vi "Controller Test Bench (11).vi"() -> ()   [LabVIEW 2022 SP3]
uses:
  WhiteNoise.ctl
  <vilib>/sound2/lvsound2.llb/Sound Data Format.ctl
  <vilib>/Utility/error.llb/DialogType.ctl
  <vilib>/sound2/lvsound2.llb/Sampling Mode.ctl
  <vilib>/Platform/TimedLoop/XDataNode/timing_clust.ctl
  <vilib>/Platform/TimedLoop/XDataNode/nitl_modes.ctl
  <vilib>/Platform/TimedLoop/XDataNode/wakeup.ctl
  <vilib>/sound2/lvsound2.llb/Sound File Refnum.ctl
  <vilib>/Analysis/4window.llb/windowTd.ctl
  <vilib>/DAQmx/write.llb/DAQmx Write (Analog 1D Wfm NChan NSamp).vi
  <vilib>/DAQmx/read.llb/DAQmx Read (Analog 1D Wfm NChan NSamp).vi
  <vilib>/DAQmx/create/channels.llb/DAQmx Create Channel (AI-Acceleration-Accelerometer).vi
  <vilib>/DAQmx/configure/timing.llb/DAQmx Timing (Sample Clock).vi
  <vilib>/Platform/TimedLoop/scheduler/LVUserAPI/_suppVIs/Create_1kHz_TSource.vi
  <vilib>/DAQmx/create/channels.llb/DAQmx Create Channel (AO-Voltage-Basic).vi
  <vilib>/sound2/lvsound2.llb/Sound File Info (path).vi
  <vilib>/sound2/lvsound2.llb/Sound File Read Open.vi
  <vilib>/sound2/lvsound2.llb/Sound File Read (DBL).vi
  <vilib>/DAQmx/miscellaneous.llb/DAQmx Fill In Error Info.vi
  <vilib>/sound2/lvsound2.llb/Sound Output Set Volume (Single).vi
  <vilib>/sound2/lvsound2.llb/Sound Output Write (DBL).vi
  <vilib>/DAQmx/configure/task.llb/DAQmx Configure Logging (TDMS).vi
  <vilib>/measure/maspectr.llb/FFT Spectrum (Mag-Phase) for N Chan.vi
  <vilib>/platform/TimedLoop/XDataNode/XDataNode.xnode
  <vilib>/measure/NI_MAPro.lvlib
  <resource>/objmgr/daqmx.rc
  <vilib>/Analysis/NI_AALPro.lvlib
  <vilib>/measure/NI_MABase.lvlib
  <vilib>/Platform/TimedLoop/XDataNode/XDNodeRunTimeDep.lvlib
  <vilib>/addons/control/pid/NI_PID_pid.lvlib
  <vilib>/addons/control/pid/pid.llb/PID (DBL Array).vi
  <vilib>/sound2/lvsound2.llb/Sound Output Write (DBL Single).vi
panel:
  in  "Folder to save file to":path=path "C:/Users/LAV-UFSC/OneDrive - UFSC/Documents/LAV - TCC/Dados-Experimentos/Dados Bancada LABVIEW"
  in  "Time Out (s)":dbl=60.0
  out "Elapsed Time":i32 caption="Elapsed Time (s)" format="%.2f"
  in  "Time Out (s)":dbl=1000.0
  out "Active Controller Output":dbl[](graph)
  out "Elapsed Time":i32 caption="Elapsed Time (s)" format="%.2f"
  in  "Acquisition\nPeriod(ms)":dbl=41.2
  out "Accel.1":waveform(dbl)[](graph)
  out "Waveform Chart":waveform(dbl)[](graph)
  in  "Output Noise":bool=TRUE
  in  "?":T1(tab)=enum."Harmonic"
  in  "Cluster 3":T2={"Path txt/csv File"=path "C:/Users/LAV-UFSC-2023/Documents/LAV-TCC/Dados-Experimentos/acc_time/Previous Data/handlebar_acc1_run2.txt", "Delimiter"=".", "Separator"="\\t", "Offset (lines)"=21.0}
  in  "Gain":i32
  in  "Stop 3":bool
  in  "Gain":i32
  in  "Cluster 4":T4={"Seed"=0.0, "Iterator"=1.0, "Path Sound File"=path "C:/Users/LAV-UFSC-2023/Documents/LAV-TCC/Dados-Experimentos/Dados Empíricos/Uni-cheio.wav", "number of samples/ch (-1: all)"=-1}
  in  "Stop 2":bool
  in  "Cluster":T5={"Seed"=0.0, "Standard Deviation"=0.2, "Reset"=FALSE, "Iterator"=1.0, "Seed"=-1, "Stop 4"=FALSE, "Lower Cut-Off 2"=5.0, "Upper Cut-Off 2"=200.0} {"Upper Cut-Off 2" min=5.0 max=350.0 step=10.0; "Lower Cut-Off 2" min=5.0 max=350.0 step=10.0; "Standard Deviation" min=0.001 max=1.5 step=0.05 format="%0.2p"}
  in  "Cluster 2":T6={"Iterator"=1.0, "Waveform Type"=0, "Frequency"=10.0, "Amplitude"=0.25, "Stop 4"=FALSE} {"Frequency" min=5.0 max=350.0 step=10.0 format="%0.2p"; "Waveform Type" items=["Sine Wave", "Triangle Wave", "Square Wave", "Sawtooth Wave"]; "Amplitude" min=0.001 max=0.3 step=0.05 format="%0.2p"}
  in  "Active Control":bool
  in  "Tab Control":T7(tab)
  out "dt out (s)":dbl format="%.3f"
  in  "setpoint":dbl[](array[numeric])=[0.0] format="%.2f"
  in  "PID gains":T8(array[cluster])=[{"proportional gain (Kc)"=1.0, "integral time (Ti, min)"=0.01, "derivative time (Td, min)"=0.0}] {"derivative time (Td, min)" format="%.6f"; "integral time (Ti, min)" format="%.6f"; "proportional gain (Kc)" step=1e-05 format="%.6f"}
  in  "dt (s)":dbl=-1.0 format="%.3f"
  in  "output range":cluster{"output high":dbl, "output low":dbl}[](array[cluster])=[{"output high"=100.0, "output low"=-100.0}, {"output high"=3.0, "output low"=-3.0}] {"output low" format="%.2f"; "output high" format="%.2f"}
  in  "Upper Cut-Off":dbl=150.0
  in  "Lower Cut-Off":dbl=50.0
  in  "Setpoint":dbl
  in  "Gain":dbl min=0.0 step=0.01
  out "Output Signal":dynamicdata(graph)
  in  "Upper Cut-Off":dbl=400.0
  in  "Lower Cut-Off":dbl=100.0
  out "Accel.2":waveform(dbl)[](graph)
  in  "Log Raw Data":bool
  out "Phase 2":cluster{"f0":dbl, "df":dbl, "phase":dbl[]}[](graph)
  out "Mag 2":cluster{"f0":dbl, "df":dbl, "magnitude":dbl[]}[](graph)
  in  "Show FFT":bool=TRUE
  in  "Log FFT":bool
  in  "Start Reading":bool=TRUE
  in  "Stop":bool
  # "Active Controller"
  # "Main\nSwitch"
  # "Output Noise"
  # "RAW - Accel. 1"
  # "Data Acquisition"
  # "FFT - Amplitude (dB)"
  # "FFT - Phase (°)"
  # "RAW - Accel. 2"
  # "Runtime"
  # "Pre-Set"
  # "Runtime"
  # "Pre-Set"
  # "Runtime"
  # "Filter"
  # "Runtime"
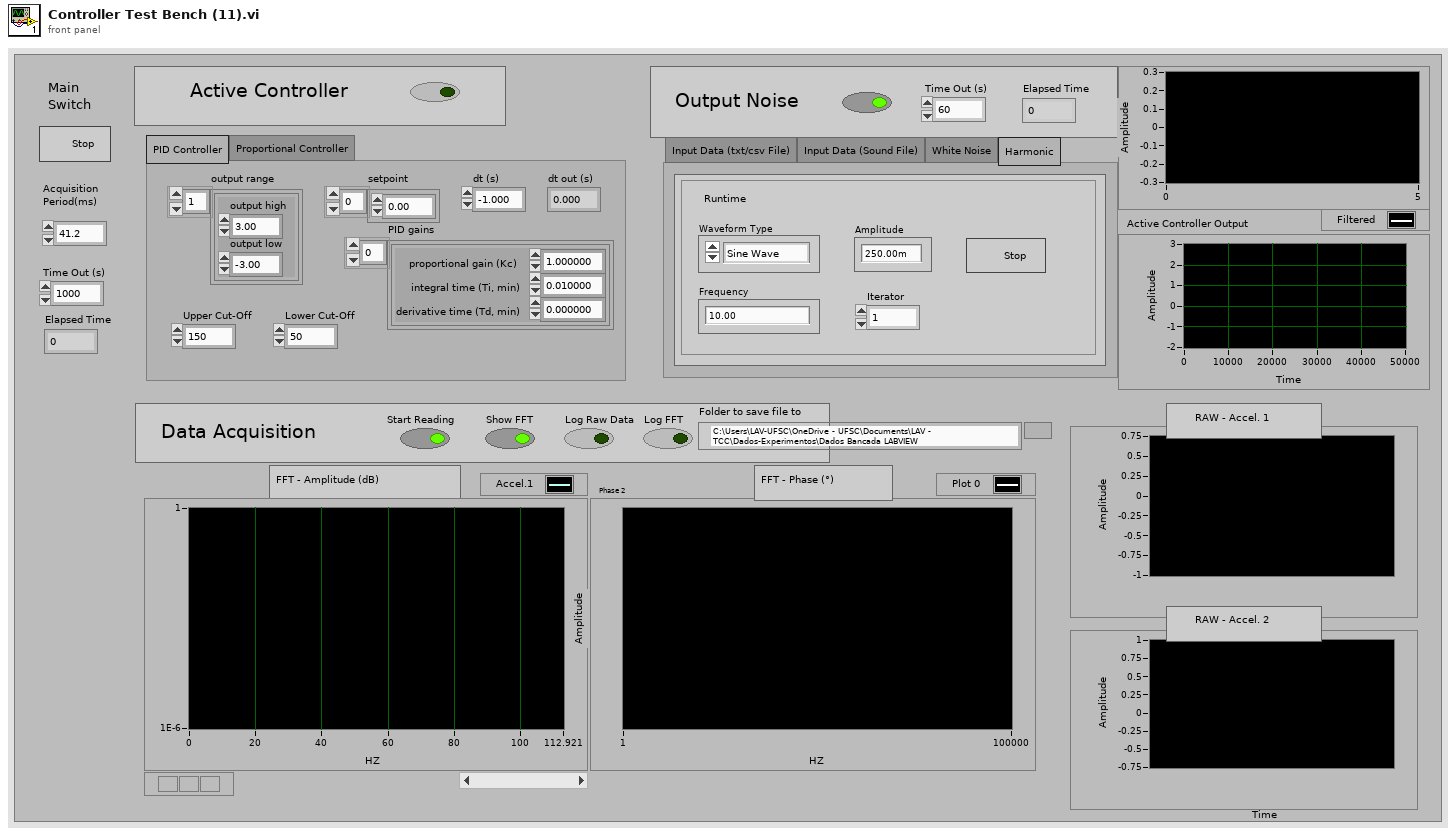
[diagram p1: front panel]
types:
  T1 = enum32{"Input Data (txt/csv File)", "Input Data (Sound File)", "White Noise", "Harmonic"}
  T2 = cluster{"Path txt/csv File":path, "Delimiter":string, "Separator":string, "Offset (lines)":dbl}
  T3 = typedef "WhiteNoise.ctl" = dbl
  T4 = cluster{"Seed":T3, "Iterator":dbl, "Path Sound File":path, "number of samples/ch (-1: all)":i32}
  T5 = cluster{"Seed":T3, "Standard Deviation":dbl, "Reset":bool, "Iterator":dbl, "Seed":i8, "Stop 4":bool, "Lower Cut-Off 2":dbl, "Upper Cut-Off 2":dbl}
  T6 = cluster{"Iterator":dbl, "Waveform Type":u16, "Frequency":dbl, "Amplitude":dbl, "Stop 4":bool}
  T7 = enum32{"PID Controller", "Proportional Controller"}
  T8 = cluster{"proportional gain (Kc)":dbl, "integral time (Ti, min)":dbl, "derivative time (Td, min)":dbl}[]
  T9 = typedef "Sampling Mode.ctl" = i32
  T10 = typedef "DialogType.ctl" = u16
  T11 = typedef "Sound Data Format.ctl" = cluster{"sample rate (S/s)":dbl, "number of channels":i32, "bits per sample":i32}
  T12 = typedef "Sound File Refnum.ctl" = refnum<file>
  T13 = typedef "XDNodeRunTimeDep.lvlib/timing_clust.ctl" = cluster{"Expected End [f-1]":u64, "Actual End [f-1]":u64, "Finished Late? [f-1]":bool, "Expected End [i-1]":u64, "Actual End [i-1]":u64, "Finished Late? [i-1]":bool, "Expected Start [i]":u64, "Actual Start [i]":u64, "Expected Start [f]":u64, "Actual Start [f]":u64, "Source Name":string, "Structure Name":string, "Period":i64, "Deadline":i64, "Offset":i64, "Start":i64, "Priority":i32, "Timeout":i32, "Mode":T14, "Wakeup Reason":T15, "Error":errorcluster, "Source Type":string, "Secondary Source Type":string, "Global End Time":u64, "Global Start Time":u64, "Frame Duration":u64, "Iteration Duration":u64, "Assigned CPU":i32, "I/O Scan Engine Mode":u32}
  T14 = typedef "XDNodeRunTimeDep.lvlib/nitl_modes.ctl" = enum32{"No Change", "Process missed periods, maintain original phase", "Discard missed periods, maintain original phase", "Process missed periods, ignore original phase", "Discard missed periods, ignore original phase"}
  T15 = typedef "XDNodeRunTimeDep.lvlib/wakeup.ctl" = enum32{"Normal", "Aborted", "Asynchronous wakeup", "Timing source error", "Timed loop error", "Timeout"}
  T16 = typedef "Sound Output Task ID.ctl" = u32
  T17 = typedef "NI_AALPro.lvlib/windowTd.ctl" = u32
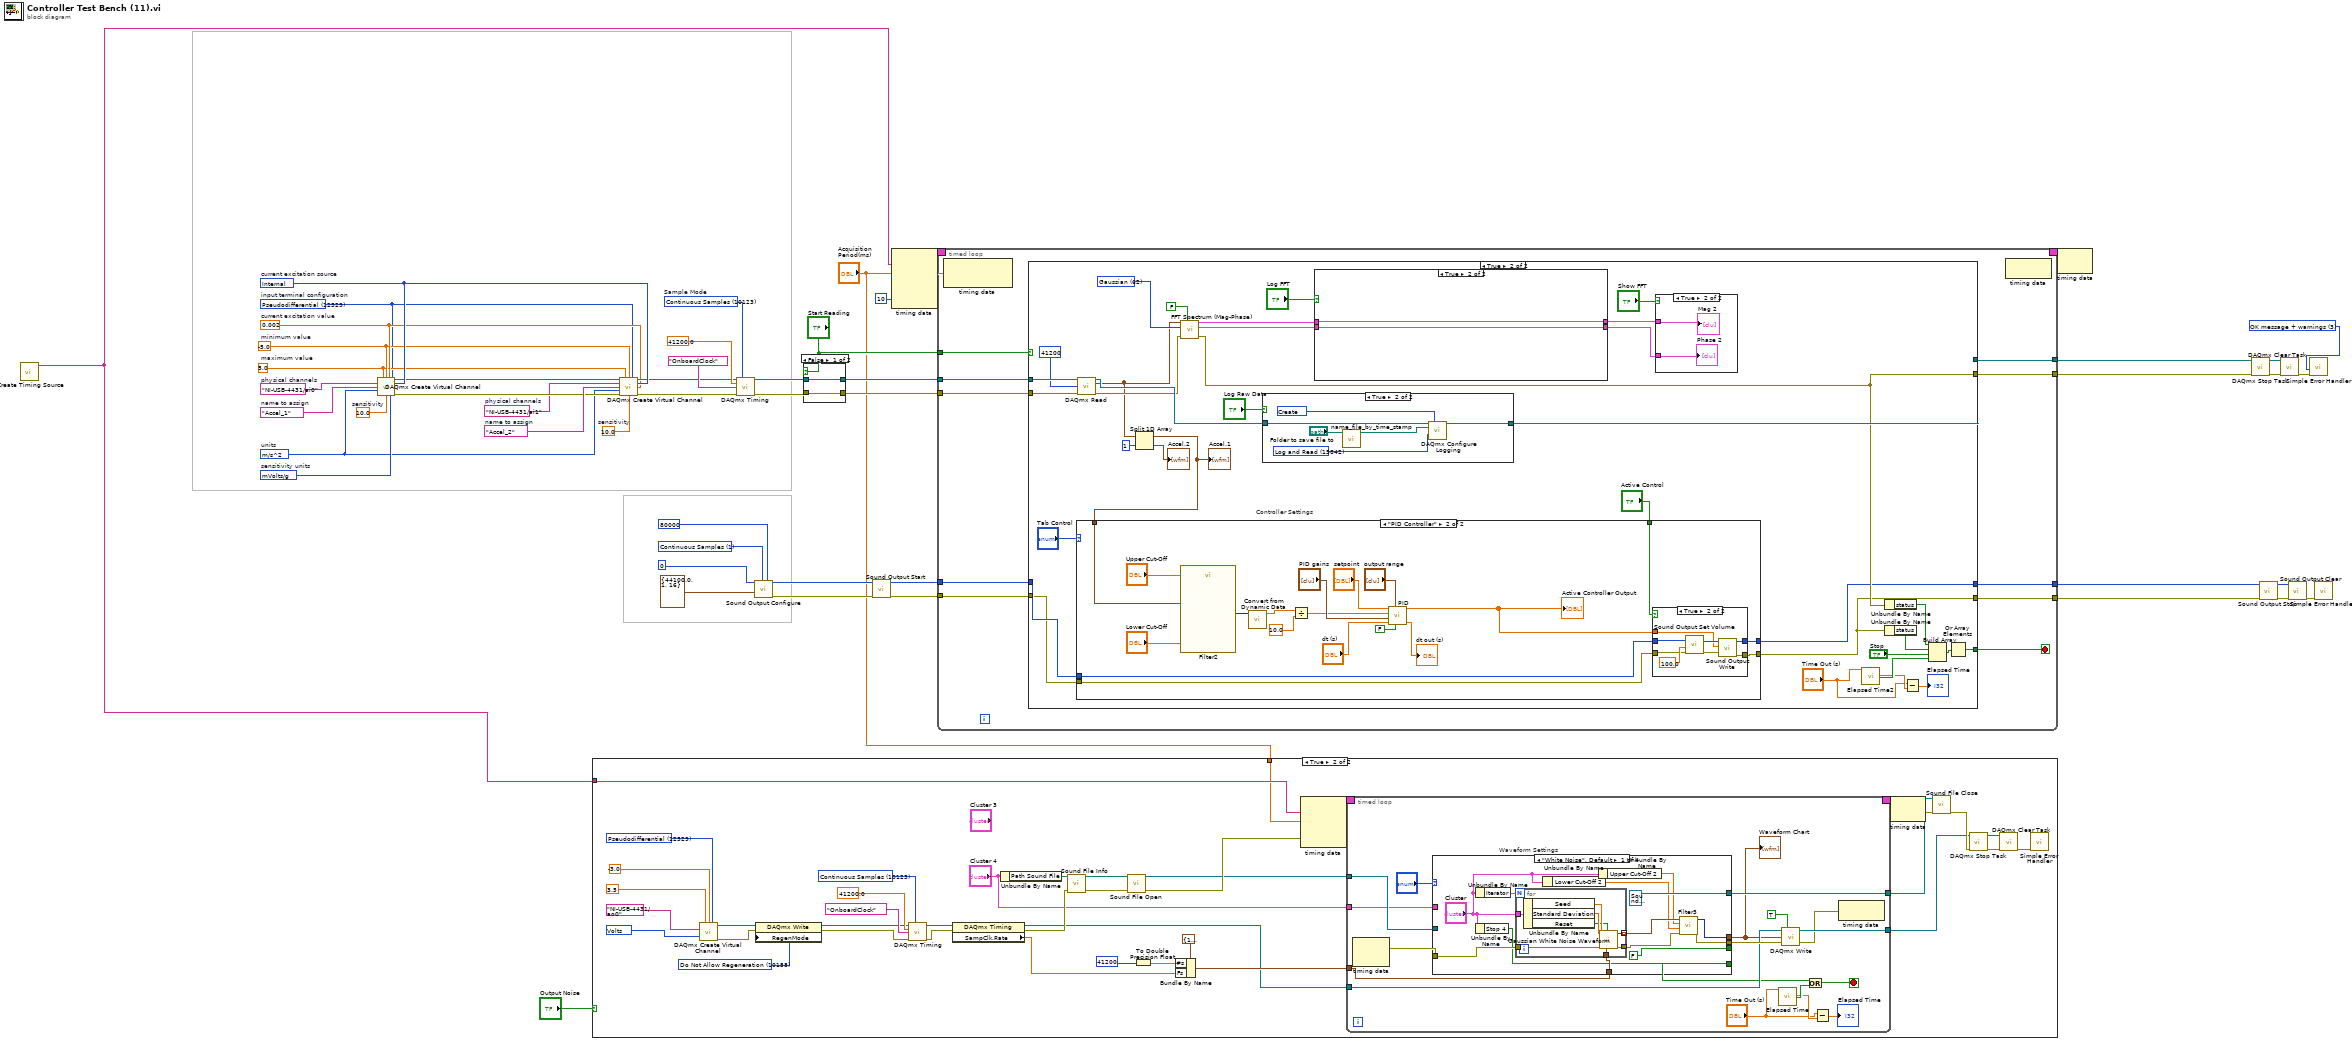
[diagram p0: block diagram]
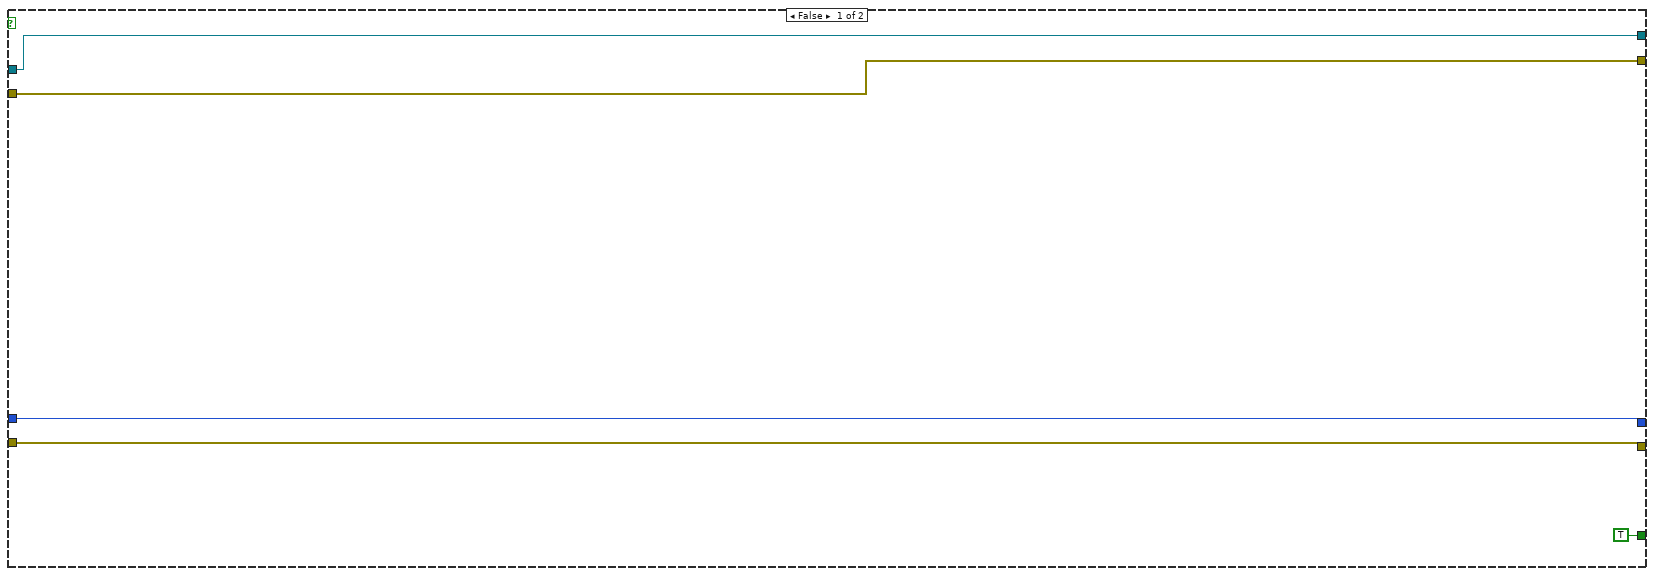
[diagram p2: hidden frame]
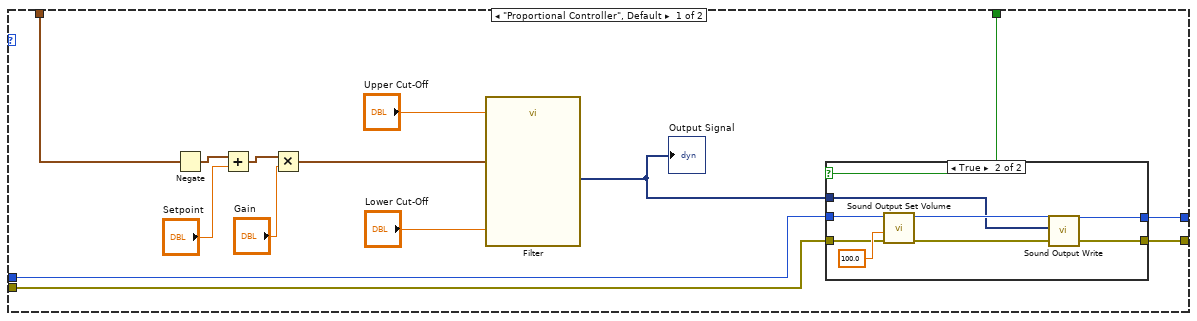
[diagram p3: hidden frame]
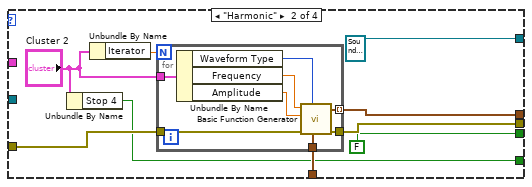
[diagram p10: hidden frame]
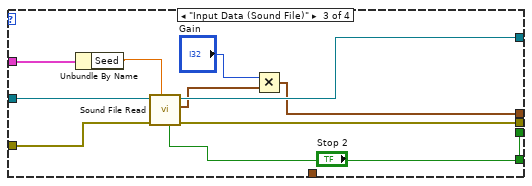
[diagram p11: hidden frame]
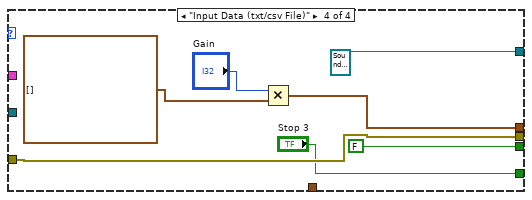
[diagram p12: hidden frame]
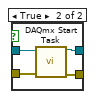
[diagram p13: hidden frame]
diagram:
  w38 = 12509 items=["mVolts/g"=12509, "Volts/g"=12510]  # sensitivity units
  w39 = 10.0  # sensitivity
  w29 = 0.002  # current excitation value
  w32 = 10200 items=["Internal"=10200, "External"=10167, "None"=10230]  # current excitation source
  w22 = tag "NI-USB-4431/ai0"  # physical channels
  w37 = 10123 items=["Finite Samples"=10178, "Continuous Samples"=10123, "Hardware Timed Single Point"=12522]  # Sample Mode
  w25 = 12529 items=["default"=-1, "RSE"=10083, "NRSE"=10078, "Differential"=10106, "Pseudodifferential"=12529]  # input terminal configuration
  w28 = -5.0  # minimum value
  w27 = 5.0  # maximum value
  w40 = "Accel_1"  # name to assign
  w26 = 12470 items=["g"=10186, "m/s^2"=12470, "in/s^2"=12471, "From Custom Scale"=10065]  # units
  w41 = 10.0  # sensitivity
  w23 = tag "NI-USB-4431/ai1"  # physical channels
  w34 = "Accel_2"  # name to assign
  w42 = T9 1 items=["Finite Samples", "Continuous Samples"] ("sample mode")
  w43 = T10 3 items=["no dialog", "OK message", "continue or stop message", "OK message + warnings", "continue/stop + warnings"] ("type of dialog (OK msg:1)")
  n1 = call-poly <vilib>:"Create Timing Source.vi"() -> ("name (out)"=w11:string)  [unwired: 10 in, 1 out]
  n2 = call-poly <vilib>:"DAQmx Create Virtual Channel.vi"("maximum value"=w27, "minimum value"=w28, "input terminal configuration"=w25, "physical channels"=w22, "current excitation source"=w32, "name to assign"=w40, "current excitation value"=w29, "units"=w26, "sensitivity"=w39, "sensitivity units"=w38) -> ("task out"=w24:refnum<k21>, "error out"=w33:errorcluster)  [unwired: 4 in]
  n3 = case shown="True" "Output Noise" {
    tunnel: w11 -> [_ w61]
    tunnel: "Acquisition\nPeriod(ms)" -> [_ w51]
    frame False {
    }
    frame True {
      w77 = 10123 items=["Finite Samples"=10178, "Continuous Samples"=10123, "Hardware Timed Single Point"=12522] ("sample mode")
      w81 = 10158 items=["Allow Regeneration"=10097, "Do Not Allow Regeneration"=10158] ("RegenMode")
      w87 = 12529 items=["Default"=-1, "RSE"=10083, "Differential"=10106, "Pseudodifferential"=12529] ("output terminal configuration")
      w85 = 10348 items=["Volts"=10348, "From Custom Scale"=10065] ("units")
      n4 = call-poly <vilib>:"DAQmx Create Virtual Channel.vi"("maximum value"=3.5, "minimum value"=-3.0, "output terminal configuration"=w87, "physical channels"=tag "NI-USB-4431/ao0", "units"=w85) -> ("task out"=w80:refnum<k21>, "error out"=w82:errorcluster)  [unwired: 9 in]
      n5 = property class="DAQmx Write"(reference=w80, error in=w82, "RegenMode"=w81) -> (reference out=w78:refnum<k21>, error out=w79:errorcluster)
      n6 = call-poly <vilib>:"DAQmx Timing.vi"("task/channels in"=w78, "sample mode"=w77, "rate"=41200.0 ("Sample Rate"), "source"=tag "OnboardClock" ("Sample Clock Source"), "error in"=w79) -> ("task out"=w73:refnum<k21>, "error out"=w72:errorcluster)  [unwired: 9 in]
      n7 = property class="DAQmx Timing"(reference=w73, error in=w72) -> (reference out=w56:refnum<k21>, error out=w66:errorcluster, "SampClk.Rate"=w74:dbl)
      n8 = Unbundle By Name("Cluster 4") -> ("Path Sound File"=w54:path)
      n9 = call-poly <vilib>:"Sound File Info.vi"("error in (no error)"=w66, "path"=w54) -> ("error out"=w68:errorcluster, "path out"=w67:path)  [unwired: 6 in, 2 out]
      n10 = call-poly <vilib>:"Sound File Open.vi"("error in (no error)"=w68, "path"=w67) -> ("error out"=w62:errorcluster, "sound file refnum"=w60:T12)  [unwired: 8 in]
      n11 = To Double Precision Float(number=41200) -> (double precision float=w75:dbl)
      n12 = Bundle By Name(cluster=cluster{"Fs":dbl, "#s":dbl} {"Fs"=1000.0, "#s"=1000.0} ("sampling info"), "#s"=w75, "Fs"=w74) -> (w57:cluster{"Fs":dbl, "#s":dbl})
      n13 = node-c288(w61, w51, w62) -> (w64:T13)  [unwired: 1 in]
      n14 = timed-loop {
        timing: w64 -> [_]
        timing-out: [_] -> w63
        tunnel: w60 -> [w103]
        tunnel: [w102] -> w59
        tunnel: [w101] -> w58
        tunnel: w57 -> [w100]
        tunnel: w56 -> [w99]
        tunnel: "Cluster 4" -> [w98]
        stop <- w96 stop-if-true
        # "Waveform Settings"
        n15 = node-c288() -> (w104:errorcluster)  [unwired: 1 in, 1 out]
        n16 = case shown="\"White Noise\", Default" "?" {
          tunnel: w100 -> [w120 w135 _ _]
          tunnel: w104 -> [w118 w137 w156 w161]
          tunnel: [w111 w134 w155 w161] -> w106
          tunnel: [w113 w136 w151 w157] -> w97
          tunnel: w103 -> [_ _ w154 _]
          tunnel: [FALSE FALSE w153 FALSE ("end of file?")] -> _
          tunnel: [T12 refnum ("sound file refnum out") T12 refnum ("sound file refnum out") w152 T12 refnum ("sound file refnum out")] -> w102
          tunnel: w98 -> [_ _ w148 _]
          tunnel: [w115 w129 "Stop 2" "Stop 3"] -> w95
          frame "White Noise", Default {
            n17 = Unbundle By Name("Cluster") -> ("Iterator"=w119:dbl)
            n18 = Unbundle By Name("Cluster") -> ("Stop 4"=w115:bool)
            n19 = for {
              N: w119 -> [_]
              tunnel: w118 -> [w128]
              tunnel: w120 -> [w127]
              tunnel: [w126] -> w112
              tunnel: "Cluster" -> [w125]
              tunnel: [w124] -> w114 mode=indexing
              n20 = Unbundle By Name(w125) -> ("Seed"=w123:T3, "Standard Deviation"=w122:dbl, "Reset"=w121:bool)
              n21 = call <vilib>:"Gaussian White Noise Waveform.vi"("sampling info"=w127, "reset signal"=w121, "error in (no error)"=w128, "seed"=w123, "standard deviation"=w122) -> ("error out"=w126:errorcluster, "signal out"=w124:waveform(dbl))  [unwired: 5 in]
            }
            n22 = Unbundle By Name("Cluster") -> ("Lower Cut-Off 2"=w109:dbl)
            n23 = Unbundle By Name("Cluster") -> ("Upper Cut-Off 2"=w108:dbl)
            n24 = call "Filter3"("error in (no error)"=w112, "Lower Cut-Off"=w109, "Upper Cut-Off"=w108, "Signal"=w114) -> ("error out"=w111:errorcluster, "Filtered Signal"=w113:dynamicdata)  [unwired: 6 in]
          }
          frame "Harmonic" {
            n25 = Unbundle By Name("Cluster 2") -> ("Stop 4"=w129:bool)
            n26 = Unbundle By Name("Cluster 2") -> ("Iterator"=w133:dbl)
            n27 = for {
              N: w133 -> [_]
              tunnel: w137 -> [w145]
              tunnel: w135 -> [w144]
              tunnel: [w143] -> w134
              tunnel: "Cluster 2" -> [w142]
              tunnel: [w138] -> w136 mode=indexing
              n28 = Unbundle By Name(w142) -> ("Waveform Type"=w141:u16, "Frequency"=w140:dbl, "Amplitude"=w139:dbl)
              n29 = call <vilib>:"Basic Function Generator.vi"("sampling info"=w144, "signal type"=w141, "error in (no error)"=w145, "amplitude"=w139, "frequency"=w140) -> ("error out"=w143:errorcluster, "signal out"=w138:waveform(dbl))  [unwired: 4 in, 1 out]
            }
          }
          frame "Input Data (Sound File)" {
            n30 = Unbundle By Name(w148) -> ("Seed"=w149:T3)
            n31 = call-poly <vilib>:"Sound File Read.vi"("number of samples/ch (-1: all)"=w149, "error in (no error)"=w156, "sound file refnum"=w154) -> ("error out"=w155:errorcluster, "data"=w150:waveform(dbl)[], "sound file refnum out"=w152:T12, "end of file?"=w153:bool)  [unwired: 4 in, 1 out]
            n32 = Multiply(x="Gain", y=w150) -> (x*y=w151:waveform(dbl)[])
          }
          frame "Input Data (txt/csv File)" {
            n33 = Multiply(x="Gain", y=waveform(dbl)[] []) -> (x*y=w157:waveform(dbl)[])
          }
        }
        "Waveform Chart" <- w97
        n34 = call "Elapsed Time"("Time Target (s)"="Time Out (s)") -> ("Elapsed Time (s)"=w91:dbl, "Time has Elapsed"=w92:bool)  [unwired: 11 in, 6 out]
        n35 = call-poly <vilib>:"DAQmx Write.vi"("task/channels in"=w99, "auto start"=TRUE, "data"=w97, "error in"=w106) -> ("task out"=w101:refnum<k21>, "error out"=w94:errorcluster)  [unwired: 9 in, 1 out]
        n36 = Or(x=w95, y=w92) -> (x .or. y?=w96:bool)
        n37 = Subtract(x="Time Out (s)", y=w91) -> (x-y=→"Elapsed Time":dbl)
        n38 = node-c288(w94) -> ()  [unwired: 1 out]
      }
      n39 = node-c288(w63) -> (w52:errorcluster)
      n40 = call <vilib>:"Sound File Close.vi"("error in (no error)"=w52, "sound file refnum"=w59) -> ("error out"=w65:errorcluster)  [unwired: 9 in]
      n41 = call <vilib>:"DAQmx Stop Task.vi"("task/channels in"=w58, "error in"=w65) -> ("task out"=w71:refnum<k21>, "error out"=w70:errorcluster)  [unwired: 12 in]
      n42 = call <vilib>:"DAQmx Clear Task.vi"("task in"=w71, "error in"=w70) -> ("error out"=w69:errorcluster)  [unwired: 13 in]
      n43 = call <vilib>:"Simple Error Handler.vi"("error in (no error)"=w69) -> ()  [unwired: 4 in, 5 out]
    }
  }
  n44 = call-poly <vilib>:"DAQmx Create Virtual Channel.vi"("task in"=w24, "maximum value"=w27, "minimum value"=w28, "input terminal configuration"=w25, "physical channels"=w23, "current excitation source"=w32, "name to assign"=w34, "current excitation value"=w29, "units"=w26, "error in"=w33, "sensitivity"=w41) -> ("task out"=w31:refnum<k21>, "error out"=w30:errorcluster)  [unwired: 3 in]
  n45 = call-poly <vilib>:"DAQmx Timing.vi"("task/channels in"=w31, "sample mode"=w37, "rate"=41200.0 ("Sample Rate"), "source"=tag "OnboardClock" ("Sample Clock Source"), "error in"=w30) -> ("task out"=w20:refnum<k21>, "error out"=w21:errorcluster)  [unwired: 9 in]
  n46 = call <vilib>:"Sound Output Configure.vi"("number of samples/ch"=80000 ("Number of Samples/ch"), "sample mode"=w42, "sound format"=T11 {"sample rate (S/s)"=44100.0, "number of channels"=1, "bits per sample"=16} ("Sound Format"), "device ID"=u32 0 ("Device ID")) -> ("error out"=w16:errorcluster, "task ID"=w15:T16)  [unwired: 6 in]
  n47 = case shown="False" "Start Reading" {
    tunnel: w21 -> [w176 w181]
    tunnel: w20 -> [w177 w180]
    tunnel: [w177 w179] -> w7
    tunnel: [w176 w178] -> w8
    frame False {
    }
    frame True {
      n48 = call <vilib>:"DAQmx Start Task.vi"("task/channels in"=w180, "error in"=w181) -> ("task out"=w179:refnum<k21>, "error out"=w178:errorcluster)  [unwired: 12 in]
    }
  }
  n49 = call <vilib>:"Sound Output Start.vi"("error in (no error)"=w16, "task ID"=w15) -> ("error out"=w9:errorcluster, "task ID out"=w10:T16)  [unwired: 8 in]
  n50 = node-c288(w11, "Acquisition\nPeriod(ms)", i64 10 ("Offset")) -> (w13:T13)  [unwired: 2 in]
  n51 = timed-loop {
    timing: w13 -> [_]
    timing-out: [_] -> w12
    tunnel: "Start Reading" -> [w191]
    tunnel: w10 -> [w190]
    tunnel: w9 -> [w189]
    tunnel: w8 -> [w188]
    tunnel: w7 -> [w187]
    tunnel: [w186] -> w6
    tunnel: [w185] -> w5
    tunnel: [w184] -> w4
    tunnel: [w183] -> w3
    stop <- w182 stop-if-true
    n52 = node-c288() -> ()  [unwired: 1 in, 2 out]
    n53 = case shown="True" w191 {
      tunnel: w187 -> [w196 w231]
      tunnel: w188 -> [w195 w230]
      tunnel: [w196 w227] -> w185
      tunnel: [w195 w215] -> w186
      tunnel: w190 -> [w193 w208]
      tunnel: w189 -> [w194 w207]
      tunnel: [w193 w204] -> w184
      tunnel: [w194 w205] -> w183
      tunnel: [TRUE w201] -> w182
      frame False {
      }
      frame True {
        w214 = T17 62 items=["Rectangle"=0, "Hanning"=1, "Hamming"=2, "Blackman-Harris"=3, "Exact Blackman"=4, "Blackman"=5, "Flat Top"=6, "4 Term B-Harris "=7, "7 Term B-Harris"=8, "Low Sidelobe"=9, "Blackman Nuttall"=11, "Triangle"=30, "Bartlett-Hanning"=31, "Bohman"=32, "Parzen"=33, "Welch"=34, "Kaiser"=60, "Dolph-Chebyshev"=61, "Gaussian"=62] ("window")
        # "Controller Settings"
        n54 = call-poly <vilib>:"DAQmx Read.vi"("task/channels in"=w231, "number of samples per channel"=41200, "error in"=w230) -> ("task out"=w228:refnum<k21>, "data"=w203:waveform(dbl)[], "error out"=w216:errorcluster)  [unwired: 10 in]
        n55 = Split 1D Array(array=w203, index=1) -> (first subarray=w202:waveform(dbl)[], second subarray=→"Accel.2":waveform(dbl)[])
        "Accel.1" <- w202
        n56 = case shown="\"PID Controller\"" "Tab Control" {
          tunnel: w202 -> [w241 w259]
          tunnel: w208 -> [w237 w269]
          tunnel: w207 -> [w238 w268]
          tunnel: "Active Control" -> [w236 w267]
          tunnel: [w240 w266] -> w204
          tunnel: [w239 w265] -> w205
          frame "Proportional Controller", Default {
            n57 = Negate(x=w241) -> (-x=w244:waveform(dbl)[])
            n58 = Add(x=w244, y="Setpoint") -> (x+y=w243:waveform(dbl)[])
            n59 = Multiply(x=w243, y="Gain") -> (x*y=w235:waveform(dbl)[])
            n60 = call "Filter"("Lower Cut-Off"="Lower Cut-Off", "Upper Cut-Off"="Upper Cut-Off", "Signal"=w235) -> ("Filtered Signal"=w234:dynamicdata)  [unwired: 7 in, 1 out]
            "Output Signal" <- w234
            n61 = case shown="True" w236 {
              tunnel: w238 -> [w247 w253]
              tunnel: [w247 w250] -> w239
              tunnel: w237 -> [w246 w254]
              tunnel: [w246 w249] -> w240
              tunnel: w234 -> [_ w248]
              frame False {
              }
              frame True {
                n62 = call-poly <vilib>:"Sound Output Set Volume.vi"("error in (no error)"=w253, "volume"=100.0, "task ID"=w254) -> ("error out"=w251:errorcluster, "task ID out"=w252:T16)  [unwired: 7 in]
                n63 = call-poly <vilib>:"Sound Output Write.vi"("error in (no error)"=w251, "data"=w248, "task ID"=w252) -> ("error out"=w250:errorcluster, "task ID out"=w249:T16)  [unwired: 7 in]
              }
            }
          }
          frame "PID Controller" {
            n64 = call "Filter2"("Lower Cut-Off"="Lower Cut-Off", "Upper Cut-Off"="Upper Cut-Off", "Signal"=w259) -> ("Filtered Signal"=w260:dynamicdata)  [unwired: 7 in, 1 out]
            n65 = call "Convert from Dynamic Data"("Dynamic Data Type"=w260) -> ("Array"=w256:dbl[])  [unwired: 3 in]
            n66 = Divide(x=w256, y=10.0) -> (x/y=w258:dbl[])
            n67 = call-poly <vilib>:"PID.vi"("reinitialize? (F)"=FALSE, "output range"="output range", "dt (s)"="dt (s)", "PID gains"="PID gains", "process variable"=w258, "setpoint"="setpoint") -> ("dt out (s)"=→"dt out (s)":dbl, "output"=w261:dbl[])  [unwired: 4 in]
            "Active Controller Output" <- w261
            n68 = case shown="True" w267 {
              tunnel: w268 -> [w276 w282]
              tunnel: [w276 w279] -> w265
              tunnel: w269 -> [w275 w283]
              tunnel: [w275 w278] -> w266
              tunnel: w261 -> [_ w277]
              frame False {
              }
              frame True {
                n69 = call-poly <vilib>:"Sound Output Set Volume.vi"("error in (no error)"=w282, "volume"=100.0, "task ID"=w283) -> ("error out"=w280:errorcluster, "task ID out"=w281:T16)  [unwired: 7 in]
                n70 = call-poly <vilib>:"Sound Output Write.vi"("error in (no error)"=w280, "data"=w277, "task ID"=w281) -> ("error out"=w279:errorcluster, "task ID out"=w278:T16)  [unwired: 7 in]
              }
            }
          }
        }
        n71 = call-poly <vilib>:"FFT Spectrum (Mag-Phase).vi"("restart averaging (F)"=FALSE, "error in (no error)"=w216, "window"=w214, "time signals"=w203) -> ("error out"=w215:errorcluster, "phases"=w221:cluster{"f0":dbl, "df":dbl, "phase":dbl[]}[], "magnitudes"=w222:cluster{"f0":dbl, "df":dbl, "magnitude":dbl[]}[])  [unwired: 3 in, 2 out]
        n72 = case shown="True" "Log Raw Data" {
          tunnel: w228 -> [w291 w294]
          tunnel: [w291 w295] -> w227
          frame False {
          }
          frame True {
            w296 = 15848 items=["Open"=10437, "Open or Create"=15846, "Create or Replace"=15847, "Create"=15848] ("operation")
            w297 = 15842 items=["Off"=10231, "Log"=15844, "Log and Read"=15842] ("logging mode")
            n73 = call "name_file_by_time_stamp.vi"("Folder to save file to"="Folder to save file to") -> ("New file path"=w293:path)  [unwired: 10 in]
            n74 = call-poly <vilib>:"DAQmx Configure Logging.vi"("task/channels in"=w294, "operation"=w296, "file path"=w293, "logging mode"=w297) -> ("task out"=w295:refnum<k21>)  [unwired: 10 in, 1 out]
          }
        }
        n75 = case shown="True" "Log FFT" {
          tunnel: w222 -> [w285 w288]
          tunnel: w221 -> [w286 w287]
          tunnel: [w286 w287] -> w220
          tunnel: [w285 w288] -> w219
          frame False {
          }
          frame True {
          }
        }
        n76 = case shown="True" "Show FFT" {
          tunnel: w219 -> [_ w290]
          tunnel: w220 -> [_ w289]
          frame False {
          }
          frame True {
            "Mag 2" <- w290
            "Phase 2" <- w289
          }
        }
        n77 = call "Elapsed Time2"("Time Target (s)"="Time Out (s)") -> ("Elapsed Time (s)"=w198:dbl, "Time has Elapsed"=w200:bool)  [unwired: 11 in, 6 out]
        n78 = Unbundle By Name(w215) -> ("status"=w212:bool)
        n79 = Unbundle By Name(w205) -> ("status"=w218:bool)
        n80 = Subtract(x="Time Out (s)", y=w198) -> (x-y=→"Elapsed Time":dbl)
        n81 = Build Array(w212, w218, "Stop", w200) -> (w225:bool[])
        n82 = Or Array Elements(Boolean array=w225) -> (logical OR=w201:bool)
      }
    }
    n83 = node-c288() -> ()  [unwired: 1 in, 1 out]
  }
  n84 = node-c288(w12) -> ()  [unwired: 1 out]
  n85 = call <vilib>:"DAQmx Stop Task.vi"("task/channels in"=w5, "error in"=w6) -> ("task out"=w46:refnum<k21>, "error out"=w45:errorcluster)  [unwired: 12 in]
  n86 = call <vilib>:"Sound Output Stop.vi"("error in (no error)"=w3, "task ID"=w4) -> ("error out"=w19:errorcluster, "task ID out"=w18:T16)  [unwired: 8 in]
  n87 = call <vilib>:"DAQmx Clear Task.vi"("task in"=w46, "error in"=w45) -> ("error out"=w47:errorcluster)  [unwired: 13 in]
  n88 = call <vilib>:"Sound Output Clear.vi"("error in (no error)"=w19, "task ID"=w18) -> ("error out"=w17:errorcluster)  [unwired: 9 in]
  n89 = call <vilib>:"Simple Error Handler.vi"("type of dialog (OK msg:1)"=w43, "error in (no error)"=w47) -> ()  [unwired: 3 in, 5 out]
  n90 = call <vilib>:"Simple Error Handler.vi"("error in (no error)"=w17) -> ()  [unwired: 4 in, 5 out]
